vi "Matches.vi"(8 "error in (no error)":errorcluster, 10 "Actual":variant, 11 "String Ends With in":refnum<class "String Ends With.lvclass">) -> (0 "error out":errorcluster, 2 "Result":bool, 3 "String Ends With out":refnum<class "String Ends With.lvclass">)   [LabVIEW 2017, in "Transparent Assertions.lvlib" / "Constraints.lvlib" / "String Ends With.lvclass"]
doc: "Evaluates the constraint for <B>Actual</B>. Returns true if the constraint is met."
uses:
  String Ends With.lvclass
  String Ends With.lvclass/String Ends With.ctl
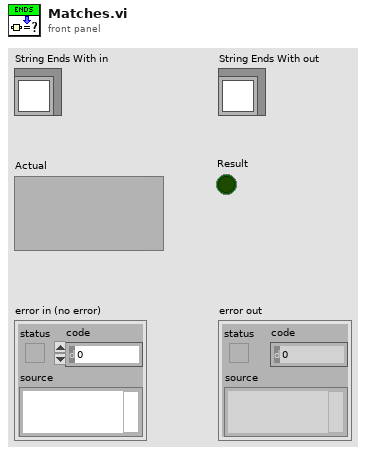
[diagram p1: front panel]
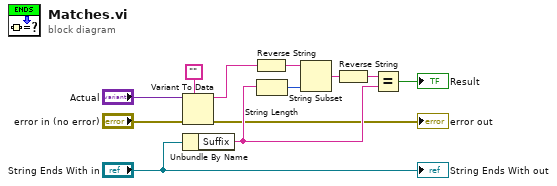
[diagram p0: block diagram]
diagram:
  n1 = Variant To Data(error in="error in (no error)", type="", Variant="Actual") -> (data=w11:string, error out=→"error out":errorcluster)
  n2 = Unbundle By Name("String Ends With in") -> ("Suffix"=w8:string)
  n3 = Reverse String(1:w11) -> (0:w2:string)
  n4 = String Length(string=w8) -> (length=w10:i32)
  n5 = String Subset(string=w2, length (rest)=w10) -> (substring=w9:string)  [unwired: 1 in]
  n6 = Reverse String(1:w9) -> (0:w1:string)
  n7 = Equal?(x=w1, y=w8) -> (x = y?=→"Result":bool)
  "String Ends With out" <- "String Ends With in"
